vi "SetSwitchTime.vi"(8 "error in":errorcluster, 10 "maxElapsedTime":cluster{"true":dbl, "false":dbl}, 11 "CRDS in":refnum<class "CRDS.lvclass">) -> (0 "error out":errorcluster, 3 "CRDS out":refnum<class "CRDS.lvclass">)   [LabVIEW 2012]
uses:
  Switch/Switch.lvclass
  CRDS.lvclass
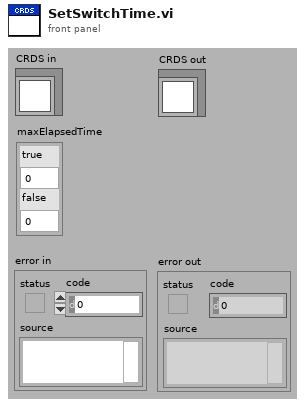
[diagram p1: front panel]
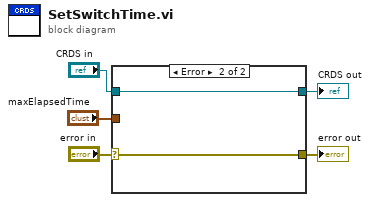
[diagram p0: block diagram]
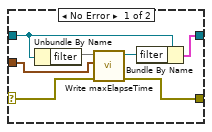
[diagram p2: hidden frame]
diagram:
  n1 = case shown="Error" "error in" {
    selector: "error in" -> [w11 w14]
    tunnel: [w10 w14] -> w4
    tunnel: [w6 w13] -> w2
    tunnel: "CRDS in" -> [w8 w13]
    tunnel: "maxElapsedTime" -> [w12 _]
    frame No Error {
      n2 = Unbundle By Name(w8) -> ("filter"=w9)
      n3 = call "Write maxElapseTime.vi"("error in"=w11, "maxElapsedTime"=w12, "Switch in"=w9) -> ("error out"=w10:errorcluster, "Switch out"=w7:refnum<class "Switch.lvclass">)  [unwired: 7 in]
      n4 = Bundle By Name(cluster=w8, "filter"=w7) -> (w6:cluster{})
    }
    frame Error {
    }
  }
  "error out" <- w4
  "CRDS out" <- w2
